vi "Try Consume Token.vi"(10 "Type":T2, 11 "Pattern Parser In":T3) -> (1 "Null?":bool, 2 "Token":T1, 3 "Pattern Parser":T3)   [LabVIEW 2020, in "Stream.lvlib" / "URLPattern.lvclass"]
uses:
  URLPattern.lvclass
  Pattern Parser.ctl
  Token.ctl
  Token Type.ctl
  Pattern Part.ctl
  Pattern Part Type.ctl
  Pattern Part Modifier.ctl
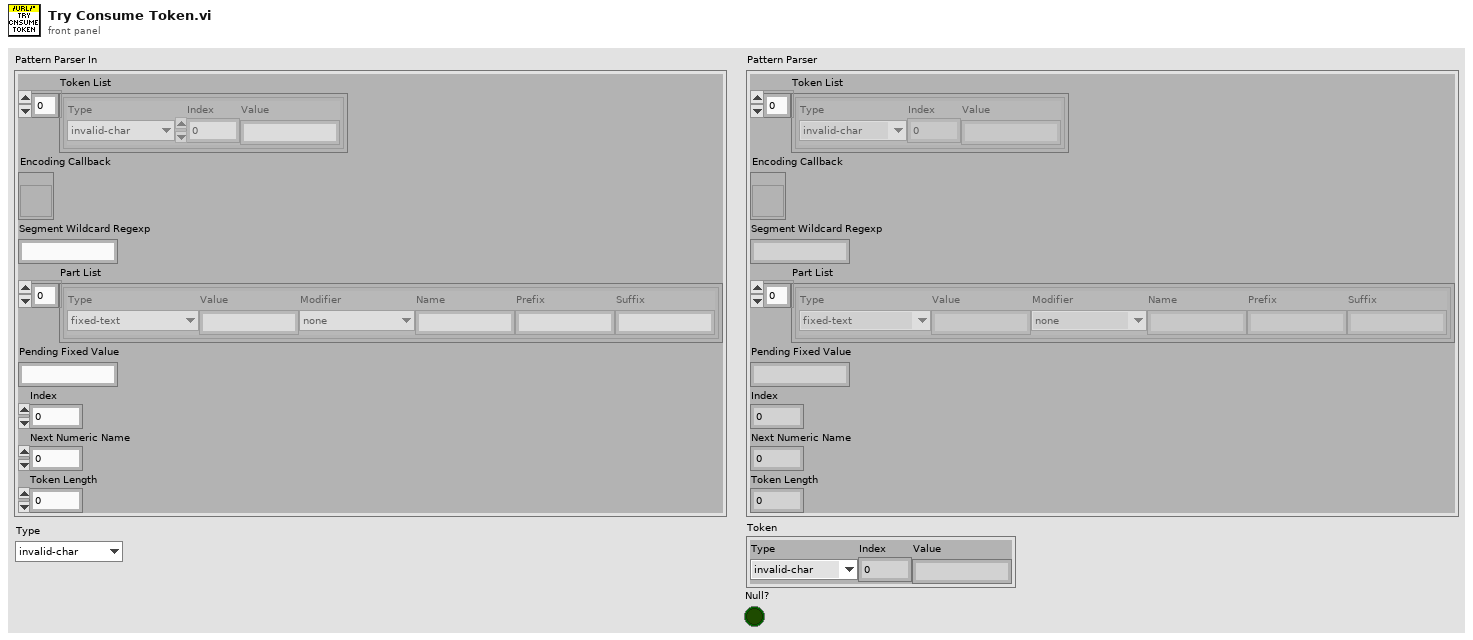
[diagram p1: front panel]
types:
  T1 = typedef "Stream.lvlib/URLPattern.lvclass/Token.ctl" = cluster{"Type":T2, "Index":i32, "Value":string}
  T2 = typedef "Stream.lvlib/URLPattern.lvclass/Token Type.ctl" = enum16{"invalid-char", "open", "close", "regexp", "name", "char", "escaped-char", "other-modifier", "asterisk", "end"}
  T3 = typedef "Stream.lvlib/URLPattern.lvclass/Pattern Parser.ctl" = cluster{"Token List":T1[], "Encoding Callback":refnum<vi>, "Segment Wildcard Regexp":string, "Part List":T4[], "Pending Fixed Value":string, "Index":i32, "Next Numeric Name":i32, "Token Length":i32}
  T4 = typedef "Stream.lvlib/URLPattern.lvclass/Pattern Part.ctl" = cluster{"Type":T5, "Value":string, "Modifier":T6, "Name":string, "Prefix":string, "Suffix":string}
  T5 = typedef "Stream.lvlib/URLPattern.lvclass/Pattern Part Type.ctl" = enum16{"fixed-text", "regexp", "segment-wildcard", "full-wildcard"}
  T6 = typedef "Stream.lvlib/URLPattern.lvclass/Pattern Part Modifier.ctl" = enum16{"none", "optional", "zero-or-more", "one-or-more"}
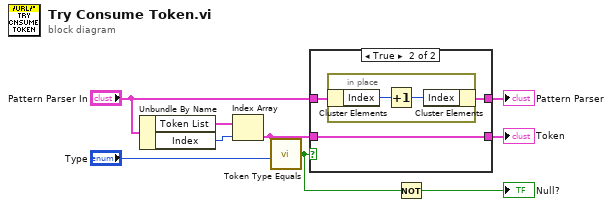
[diagram p0: block diagram]
diagram:
  n1 = Unbundle By Name("Pattern Parser In") -> ("Token List"=w9:T1[], "Index"=w8:i32)
  n2 = Index Array(array=w9, index=w8) -> (element=w5:T1)
  n3 = call "Token Type Equals.vi"("Type"="Type", "Token"=w5) -> ("Type Equals?"=w6:bool)  [unwired: 2 in]
  n4 = case shown="True" w6 {
    tunnel: w5 -> [_ w13]
    tunnel: "Pattern Parser In" -> [w10 w12]
    tunnel: [_ w13] -> w3
    tunnel: [w10 w11] -> w2
    frame False {
    }
    frame True {
      n5 = in-place {
        n6 = in-place-cluster #1(w12) -> ("Index"=w15:i32)
        n7 = Increment(x=w15) -> (x+1=w14:i32)
        n8 = in-place-cluster #1("Index"=w14) -> (w11:T3)
      }
    }
  }
  "Pattern Parser" <- w2
  "Token" <- w3
  n9 = Not(x=w6) -> (.not. x?=→"Null?":bool)
